vi "04-事件结构.vi"() -> ()   [LabVIEW 2025]
panel:
  out "Numeric":dbl
  in  "事件结构测试":bool
  out "while计数 2":i32
  out "Boolean":bool
  out "while计数":i32
  out "Waveform Chart 2":dbl(graph)
  out "次数":i32
  out "Waveform Chart":dbl(graph)
  # "到50，灯亮\n到100，弹出“到100了”\n到150，停止循环"
  # "按钮按下去的时候，\n做一件事情"
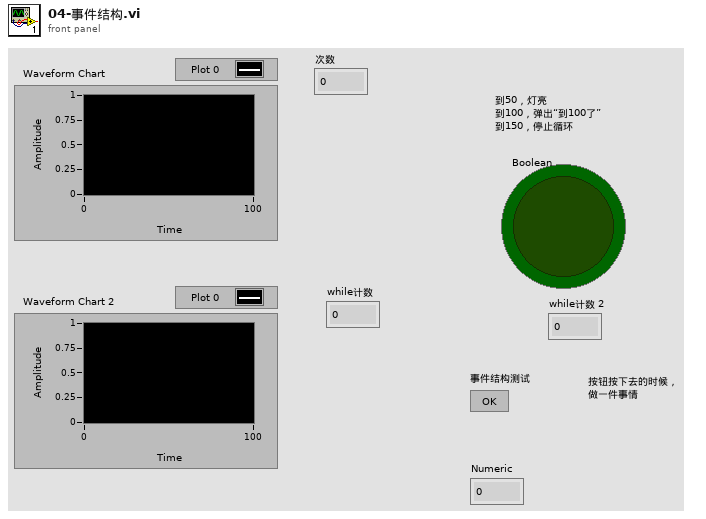
[diagram p1: front panel]
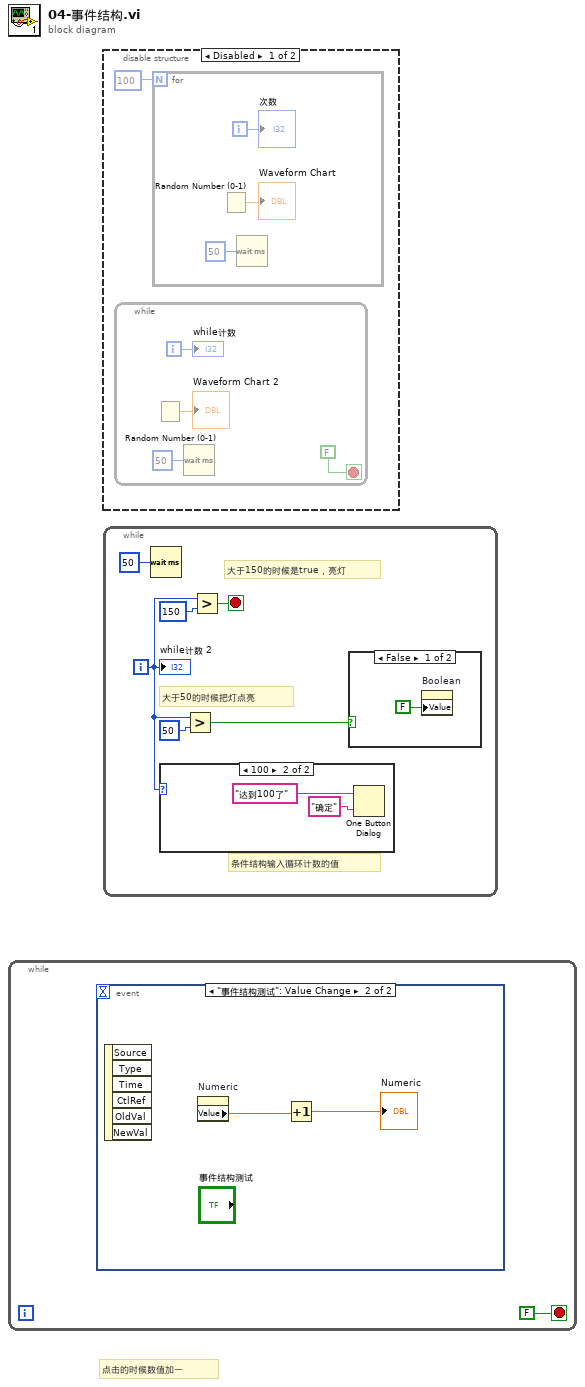
[diagram p0: block diagram]
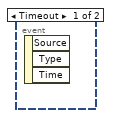
[diagram p2: hidden frame]
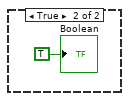
[diagram p5: hidden frame]
diagram:
  # "点击的时候数值加一"
  n1 = while {
    stop <- FALSE stop-if-true
    n2 = event shown="[1] \"事件结构测试\": Value Change" {
      selector: _ -> [_ _]
      dyn-events: _ -> [_ _]
      timeout: _ -> [_ _]
      event Timeout {
        n3 = event-data() -> ()  [unwired: 1 in, 3 out]
      }
      event "事件结构测试": Value Change {
        n4 = event-data() -> ()  [unwired: 1 in, 6 out]
        n5 = property on="Numeric" class="DigNum (strict)"() -> ("Value"=w3:dbl)  [unwired: 2 in, 2 out]
        n6 = Increment(x=w3) -> (x+1=→"Numeric":dbl)
      }
    }
  }
  n7 = disable-structure shown="Disabled" {
    frame Disabled {
      n8 = while {
        i -> [w7]
        stop <- FALSE stop-if-true
        n9 = Random Number (0-1)() -> (number: 0 to 1=→"Waveform Chart 2":dbl)
        n10 = Wait (ms)(milliseconds to wait=u32 50) -> ()  [unwired: 1 out]
        "while计数" <- w7
      }
      n11 = for {
        N: 100 -> [_]
        i -> [w9]
        n12 = Random Number (0-1)() -> (number: 0 to 1=→"Waveform Chart":dbl)
        n13 = Wait (ms)(milliseconds to wait=u32 50) -> ()  [unwired: 1 out]
        "次数" <- w9
      }
    }
    frame Enabled {
    }
  }
  n14 = while {
    i -> [w14]
    stop <- w12 stop-if-true
    # "大于150的时候是true，亮灯"
    # "条件结构输入循环计数的值"
    # "大于50的时候把灯点亮"
    n15 = Wait (ms)(milliseconds to wait=u32 50) -> ()  [unwired: 1 out]
    n16 = case shown="100" w14 {
      frame 0, Default {
      }
      frame 100 {
        n17 = One Button Dialog(message="达到100了", button name ("OK")="确定") -> ()  [unwired: 1 out]
      }
    }
    n18 = Greater?(x=w14, y=50) -> (0:w16:bool)
    n19 = Greater?(x=w14, y=150) -> (0:w12:bool)
    n20 = case shown="False" w16 {
      frame False {
        n21 = property on="Boolean" class="Bool (strict)"("Value"=FALSE ("Boolean")) -> ()  [unwired: 2 in, 2 out]
      }
      frame True {
        "Boolean" <- TRUE ("Boolean")
      }
    }
    "while计数 2" <- w14
  }
